vi "Reports.Results JSON V1 Data to Test Result V2 JSON.vi"(8 "File Data Objs":T7[](array[typedef]), 9 "JSON V1File":path) -> (2 "error out":errorcluster, 3 "Test Result V2":T8={"Type"="TestExec Results", "Version"="2.0.0", "TestEvent"={"ProcessStep"="", "StartTime"="", "EndTime"="", "Mode"="Production", "Operator"="", "Comment"="", "Result"={"State"="", "Code"=0, "Desc"="", "Details"=""}}, "UUTInfo"={"PN"="", "SN"="", "LotNumber"="", "DateCode"="", "AltID"="", "Properties"=[], "Revision"=""}, "Station"={"Name"="", "Location"="", "ConfigID"="", "PCName"="", "Slot"=""}, "TestSequence"={"Name"="", "Setup"=[]}, "NumericData"=[], "AttributeData"=[], "DataObjs"=[]})   [LabVIEW 2018]
uses:
  Report.Result State.ctl
  Report.Result Numeric.ctl
  Report.Result Attribute.ctl
  Report.Result DataObject.ctl
  Report.Result Data JSON V2.0.0.ctl
  Report.Result Test Event.ctl
  Report.Result Test Sequence.ctl
  Report.Result Test Station.ctl
  Results/Result XML/TestResult.Facility.ctl
  Results/Result XML/TestResult.HW Item.ctl
  Results/Result XML/TestResult.SW Item.ctl
  Results/Result XML/TestResult.Station Info.ctl
  Results/Result XML/TestResult.Test Run Info.ctl
  Results/Result XML/TestResult.Test Info.ctl
  Results/Result XML/TestResult.Symptom.State.ctl
  Results/Result XML/TestResult.Symptom.ctl
  Results/Result.Measurement and Attribute Item Status.ctl
  Results/Result XML/TestResult.UUT Result.ctl
  Results/Result XML/TestResult.FullResultData.ctl
  Report.Result UUTInfo.ctl
  Report.Result Data JSON V1_0_0.ctl
  Time/Time.Format Selector.ctl
  Results/Result.Measurement Item.ctl
  Report.Result Measurement JSON Safe.ctl
  Report.Result FileDataObject.ctl
panel:
  out "Test Result V1":T1={"Type"="Test Data", "Version"="1.0.0", "TestEvent"={"SN"="", "ProcessStep"="", "StartTime"="", "EndTime"="", "Mode"="", "Operator"="", "Comment"="", "Result"={"State"="", "Code"=0, "Desc"="", "Details"=""}}, "Station"={"Name"="", "Location"="", "ConfigID"="", "PCName"="", "Slot"=""}, "TestSequence"={"Name"="", "Setup"=[]}, "NumericData"=[], "AttributeData"=[], "DataObjs"=[]}
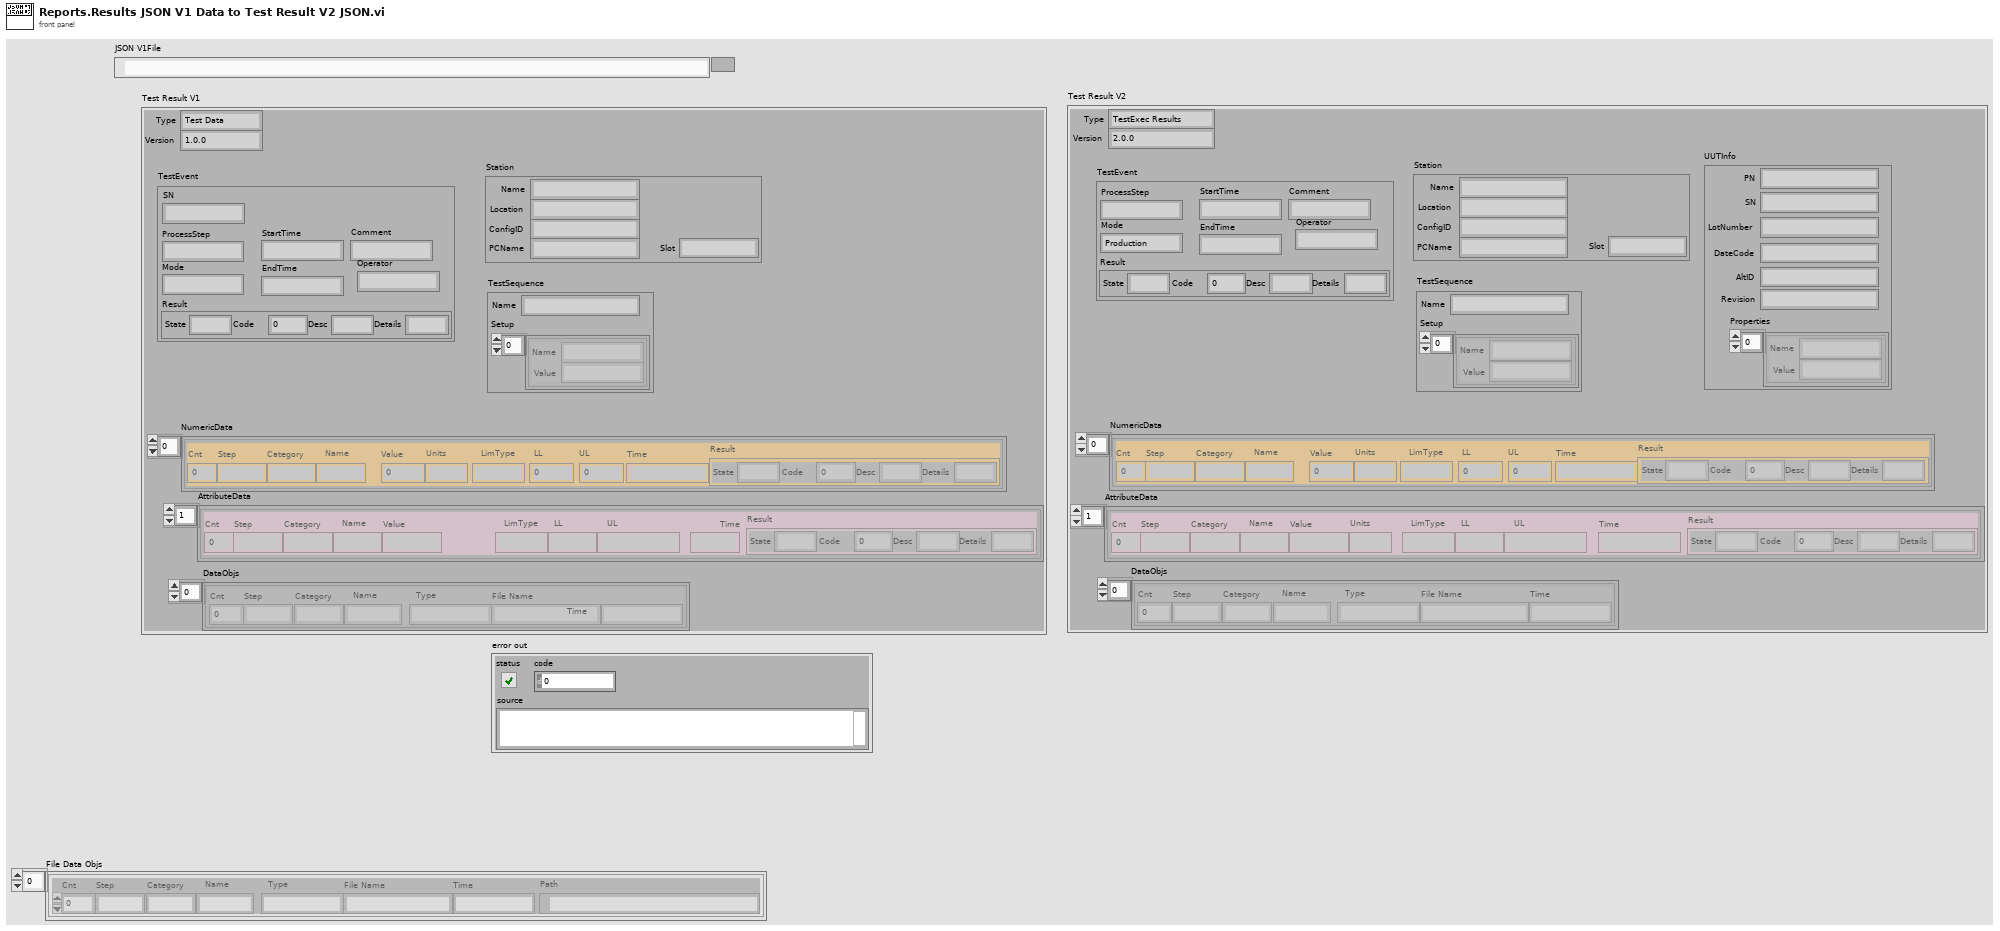
[diagram p1: front panel]
types:
  T1 = typedef "Report.Result Data JSON V1_0_0.ctl" = cluster{"Type":string, "Version":string, "TestEvent":cluster{"SN":string, "ProcessStep":string, "StartTime":string, "EndTime":string, "Mode":string, "Operator":string, "Comment":string, "Result":T2}, "Station":T3, "TestSequence":T4, "NumericData":T5[], "AttributeData":cluster{"Cnt":i32, "Step":string, "Category":string, "Name":string, "Value":string, "LimType":string, "LL":string, "UL":string, "Time":string, "Result":T2}[], "DataObjs":T6[]}
  T2 = typedef "Report.Result State.ctl" = cluster{"State":string, "Code":i32, "Desc":string, "Details":string}
  T3 = typedef "Report.Result Test Station.ctl" = cluster{"Name":string, "Location":string, "ConfigID":string, "PCName":string, "Slot":string}
  T4 = typedef "Report.Result Test Sequence.ctl" = cluster{"Name":string, "Setup":cluster{"Name":string, "Value":string}[]}
  T5 = typedef "Report.Result Numeric.ctl" = cluster{"Cnt":i32, "Step":string, "Category":string, "Name":string, "Value":dbl, "Units":string, "LimType":string, "LL":dbl, "UL":dbl, "Time":string, "Result":T2}
  T6 = typedef "Report.Result DataObject.ctl" = cluster{"Cnt":i32, "Step":string, "Category":string, "Name":string, "Type":string, "File Name":string, "Time":string}
  T7 = typedef "Report.Result FileDataObject.ctl" = cluster{"Cnt":i32, "Step":string, "Category":string, "Name":string, "Type":string, "File Name":string, "Time":string, "Path":path}
  T8 = typedef "Report.Result Data JSON V2.0.0.ctl" = cluster{"Type":string, "Version":string, "TestEvent":T9, "UUTInfo":T10, "Station":T3, "TestSequence":T4, "NumericData":T5[], "AttributeData":T11[], "DataObjs":T6[]}
  T9 = typedef "Report.Result Test Event.ctl" = cluster{"ProcessStep":string, "StartTime":string, "EndTime":string, "Mode":string, "Operator":string, "Comment":string, "Result":T2}
  T10 = typedef "Report.Result UUTInfo.ctl" = cluster{"PN":string, "SN":string, "LotNumber":string, "DateCode":string, "AltID":string, "Properties":cluster{"Name":string, "Value":string}[], "Revision":string}
  T11 = typedef "Report.Result Attribute.ctl" = cluster{"Cnt":i32, "Step":string, "Category":string, "Name":string, "Value":string, "Units":string, "LimType":string, "LL":string, "UL":string, "Time":string, "Result":T2}
  T12 = typedef "TestResult.FullResultData.ctl" = cluster{"#attributes":cluster{"Version":string}, "Facility":T13, "Station":T14, "Test Run":T17, "Test Sequence":T18, "UUTs":cluster{"UUT":T19[]}}
  T13 = typedef "TestResult.Facility.ctl" = cluster{"Name":string, "Location":string}
  T14 = typedef "TestResult.Station Info.ctl" = cluster{"Name":string, "PN":string, "SN":string, "Rev":string, "PC Name":string, "Location":string, "HW_Config":cluster{"HW_Item":T15[]}, "SW_Config":cluster{"SW_Item":T16[]}}
  T15 = typedef "TestResult.HW Item.ctl" = cluster{"Name":string, "MFG":string, "PN":string, "SN":string, "SW/FW":string, "Note":string, "Cal_ID":string, "Cal_Type":string, "Cal_Due_Date":timestamp, "Cal_Status":string}
  T16 = typedef "TestResult.SW Item.ctl" = cluster{"Name":string, "PN":string, "Version":string, "Note":string}
  T17 = typedef "TestResult.Test Run Info.ctl" = cluster{"Operator":string, "Start Time":timestamp, "Duration(s)":dbl, "Mode":string, "Comment":string, "ProcessStep":string}
  T18 = typedef "TestResult.Test Info.ctl" = cluster{"Name":string, "Config":cluster{"Config_Item":cluster{"Name":string, "Value":string}[]}}
  T19 = typedef "TestResult.UUT Info.ctl" = cluster{"Position":string, "PN":string, "SN":string, "Properties":cluster{"Property":cluster{"Name":string, "Value":string}[]}, "Result":T20, "Measurements":cluster{"Measurement":T22[]}}
  T20 = typedef "TestResult.Symptom.ctl" = cluster{"Result":T21, "Code":i32, "Description":string}
  T21 = typedef "TestResult.Symptom.State.ctl" = enum16{"Pass", "Fail", "Error", "Aborted", "Completed", "Logged"}
  T22 = typedef "Result.Measurement Item.ctl" = cluster{"Cnt":i32, "Step":string, "Category":string, "Name":string, "Value":string, "Units":string, "LimType":string, "LL":string, "UL":string, "Status":T23, "Code":i32, "Desc":string, "Time":timestamp}
  T23 = typedef "Result.Measurement and Attribute Item Status.ctl" = i32
  T24 = typedef "Time.Format Selector.ctl" = enum16{"yyyy/mm/dd HH:MM:S.sss", "yyyy-MM-ddTHH:mm:ss[.mmm]"}
  T25 = typedef "Report.Result Data JSON V2.0.0.ctl" = cluster{"Type":string, "Version":string, "TestEvent":T9, "UUTInfo":T10, "Station":T3, "TestSequence":T4, "ResultData":T26[], "DataObjs":T6[]}
  T26 = typedef "Report.Result Measurement JSON Safe.ctl" = cluster{"Cnt":i32, "Step":string, "Category":string, "Name":string, "Value":string, "Units":string, "LimType":string, "LL":string, "UL":string, "Time":string, "Result":T2}
  T27 = cluster{"SN":string, "ProcessStep":string, "StartTime":string, "EndTime":string, "Mode":string, "Operator":string, "Comment":string, "Result":T2}
  T28 = cluster{"Cnt":i32, "Step":string, "Category":string, "Name":string, "Value":string, "LimType":string, "LL":string, "UL":string, "Time":string, "Result":T2}[]
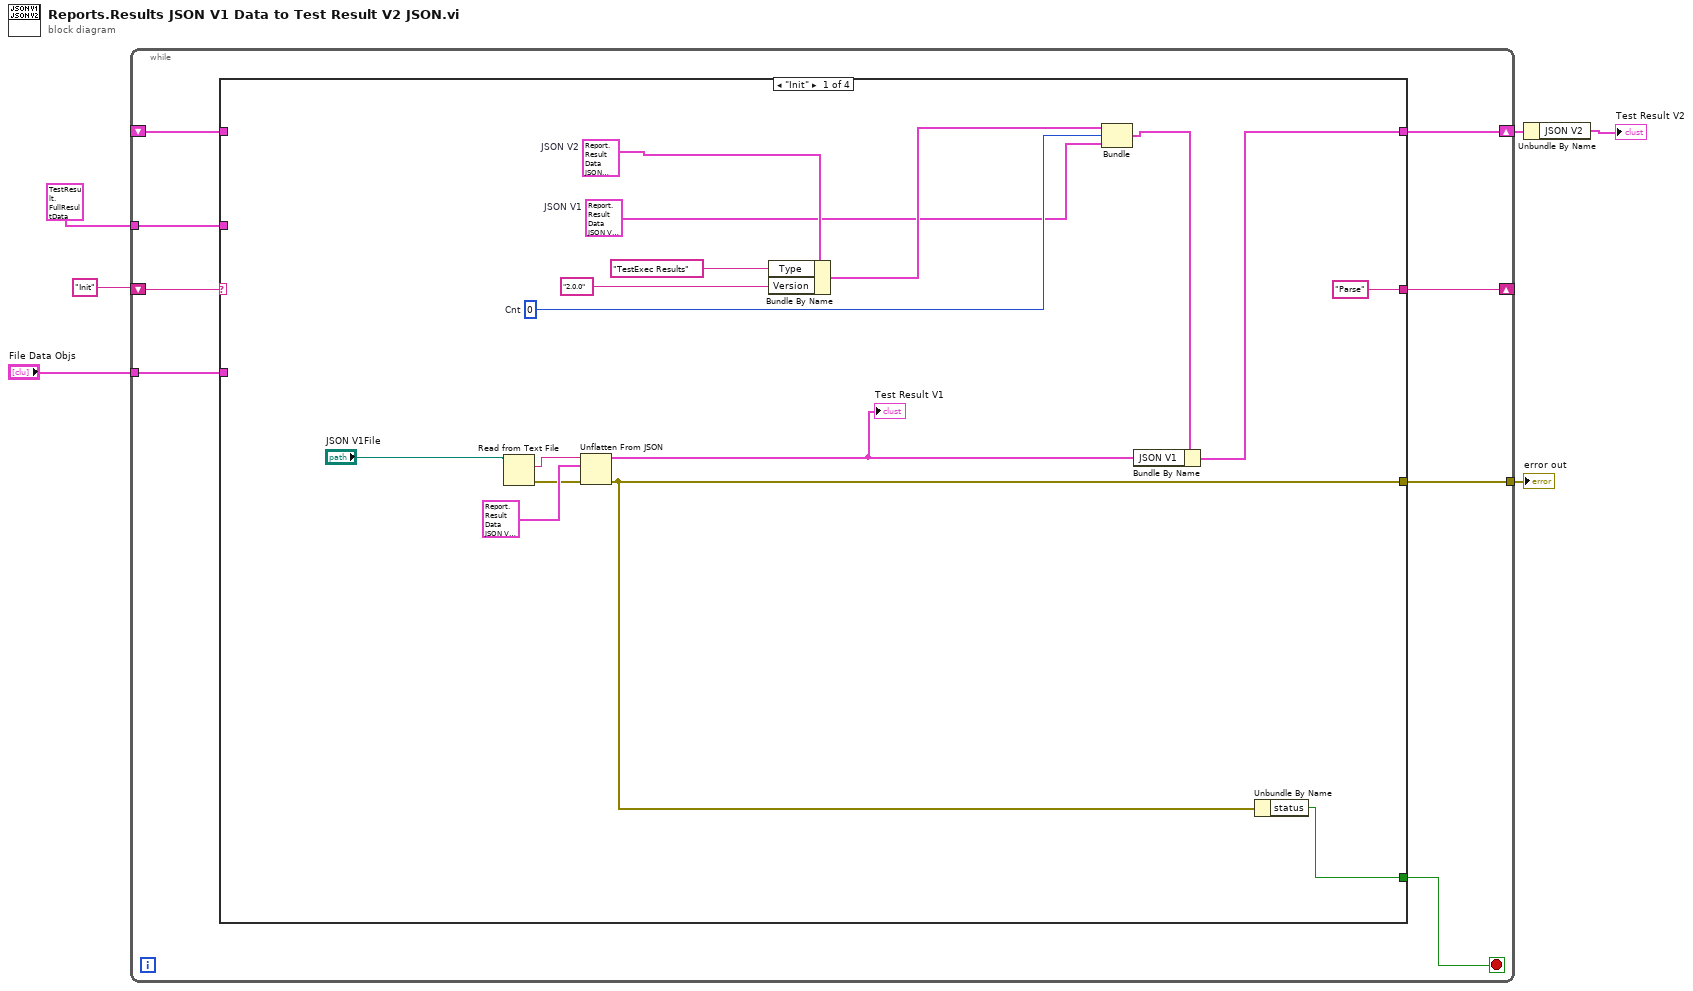
[diagram p0: block diagram]
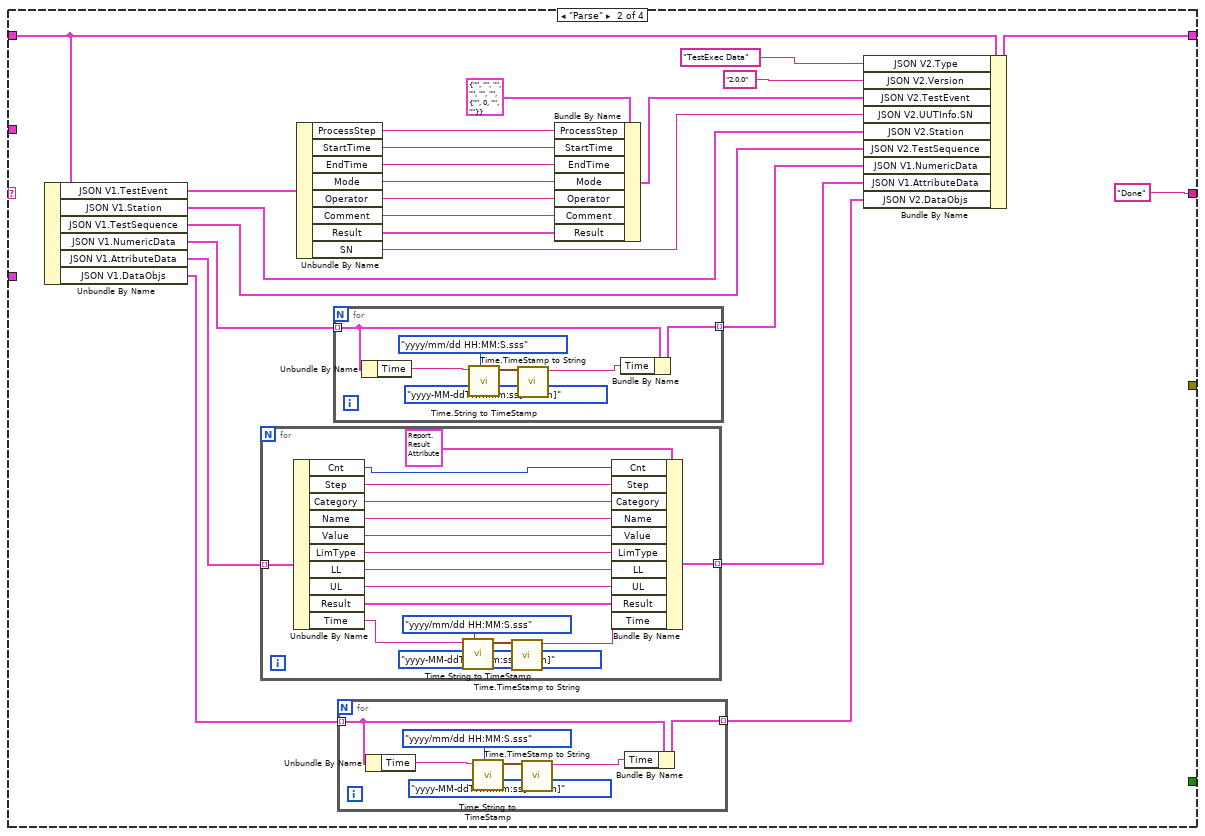
[diagram p2: hidden frame]
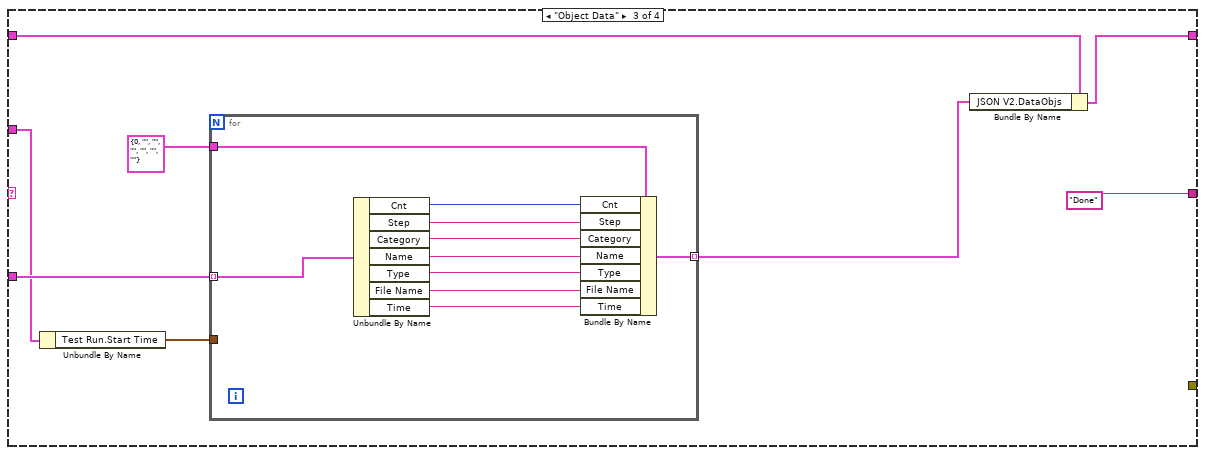
[diagram p3: hidden frame]
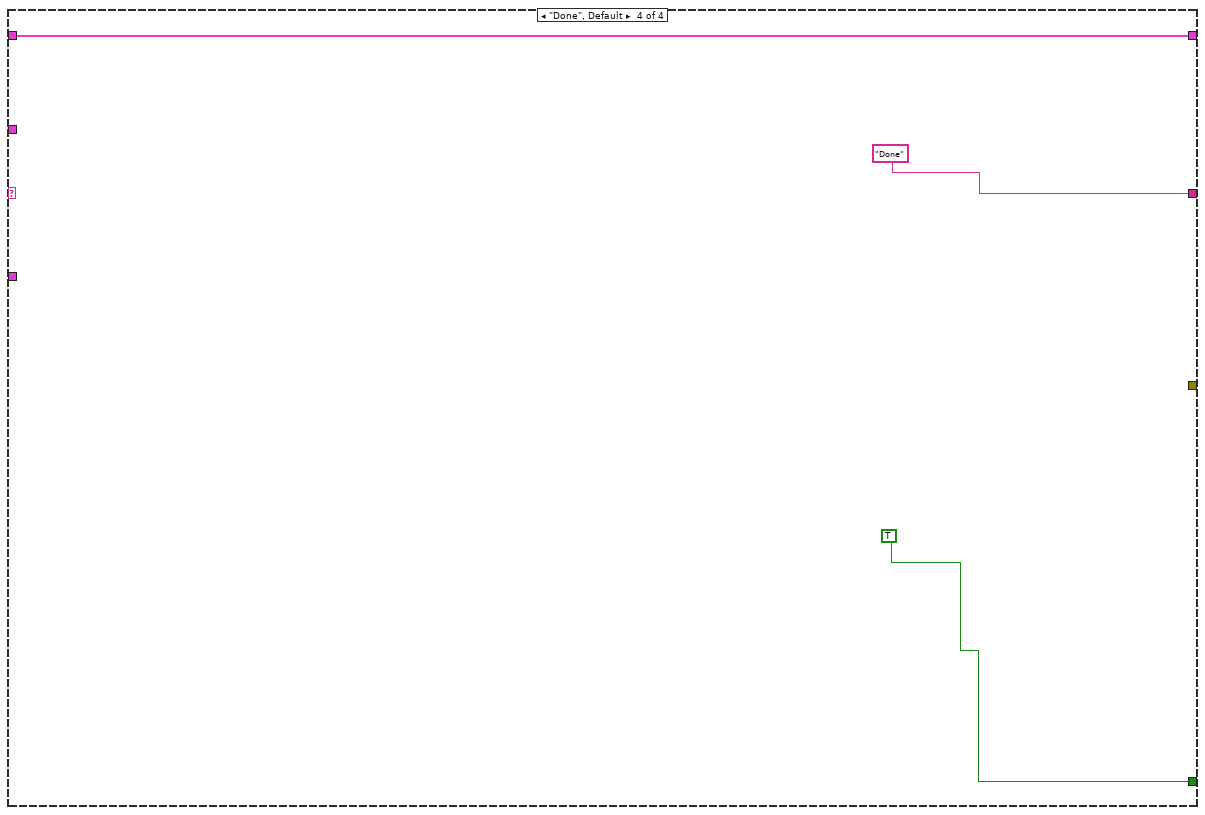
[diagram p4: hidden frame]
diagram:
  n1 = while {
    shift-right: [w8] -> w2
    shift-left: _ -> [w14]
    shift-right: [w11] -> _
    shift-left: "Init" -> [w12]
    tunnel: "File Data Objs" -> [w10]
    tunnel: T12 {"#attributes"={"Version"="MTE_1.0.0"}, "Facility"={"Name"="", "Location"=""}, "Station"={"Name"="", "PN"="", "SN"="", "Rev"="", "PC Name"="", "Location"="", "HW_Config"={"HW_Item"=[]}, "SW_Config"={"SW_Item"=[]}}, "Test Run"={"Operator"="", "Start Time"=timestamp(0 s since 1904-01-01), "Duration(s)"=0.0, "Mode"="", "Comment"="", "ProcessStep"=""}, "Test Sequence"={"Name"="", "Config"={"Config_Item"=[]}}, "UUTs"={"UUT"=[]}} ("Test Result In") -> [w9]
    tunnel: [w7] -> w1
    stop <- w13 stop-if-true
    n2 = case shown="\"Init\"" w12 {
      tunnel: w14 -> [_ w52 w87 w106]
      tunnel: [w18 w54 w93 w106] -> w8
      tunnel: [w17 _ _ TRUE] -> w13
      tunnel: ["Parse" ("Version") "Done" ("Version") "Done" ("Version") "Done"] -> w11
      tunnel: w10 -> [_ _ w89 _]
      tunnel: w9 -> [_ _ w86 _]
      tunnel: [w16 _ _ _] -> w7
      frame "Init" {
        w20 = T1 {"Type"="Test Data", "Version"="1.0.0", "TestEvent"={"SN"="", "ProcessStep"="", "StartTime"="", "EndTime"="", "Mode"="", "Operator"="", "Comment"="", "Result"={"State"="", "Code"=0, "Desc"="", "Details"=""}}, "Station"={"Name"="", "Location"="", "ConfigID"="", "PCName"="", "Slot"=""}, "TestSequence"={"Name"="", "Setup"=[]}, "NumericData"=[], "AttributeData"=[], "DataObjs"=[]}  # JSON V1
        w25 = 0  # Cnt
        w28 = T25 {"Type"="Test Data", "Version"="1.0.0", "TestEvent"={"ProcessStep"="", "StartTime"="", "EndTime"="", "Mode"="", "Operator"="", "Comment"="", "Result"={"State"="", "Code"=0, "Desc"="", "Details"=""}}, "UUTInfo"={"PN"="", "SN"="", "LotNumber"="", "DateCode"="", "AltID"="", "Properties"=[], "Revision"=""}, "Station"={"Name"="", "Location"="", "ConfigID"="", "PCName"="", "Slot"=""}, "TestSequence"={"Name"="", "Setup"=[]}, "ResultData"=[], "DataObjs"=[]}  # JSON V2
        n3 = Read from Text File(file (use dialog)="JSON V1File") -> (text=w22:string, error out=w21:errorcluster)  [unwired: 3 in, 2 out]
        n4 = Unflatten From JSON(JSON string=w22, type and defaults=T1 {"Type"="Test Data", "Version"="1.0.0", "TestEvent"={"SN"="", "ProcessStep"="", "StartTime"="", "EndTime"="", "Mode"="", "Operator"="", "Comment"="", "Result"={"State"="", "Code"=0, "Desc"="", "Details"=""}}, "Station"={"Name"="", "Location"="", "ConfigID"="", "PCName"="", "Slot"=""}, "TestSequence"={"Name"="", "Setup"=[]}, "NumericData"=[], "AttributeData"=[], "DataObjs"=[]} ("Test Result V1"), error in (no error)=w21) -> (value=w15:T1, error out=w16:errorcluster)  [unwired: 4 in]
        "Test Result V1" <- w15
        n5 = Bundle By Name(cluster=w28, "Type"="TestExec Results", "Version"="2.0.0") -> (w26:T25)
        n6 = Bundle("JSON V2"=w26, "Cnt"=w25, "JSON V1"=w20) -> (w19:cluster{"JSON V2":T25, "Cnt":i32, "JSON V1":T1})  [unwired: 1 in]
        n7 = Bundle By Name(cluster=w19, "JSON V1"=w15) -> (w18:cluster{"JSON V2":T25, "Cnt":i32, "JSON V1":T1})
        n8 = Unbundle By Name(w16) -> ("status"=w17:bool)
      }
      frame "Parse" {
        n9 = Unbundle By Name(w52) -> ("JSON V1.TestEvent"=w49:T27, "JSON V1.Station"=w38:T3, "JSON V1.TestSequence"=w37:T4, "JSON V1.NumericData"=w36:T5[], "JSON V1.AttributeData"=w34:T28, "JSON V1.DataObjs"=w33:T6[])
        n10 = for {
          tunnel: w34 -> [w78] mode=indexing
          tunnel: [w77] -> w31 mode=indexing
          n11 = Unbundle By Name(w78) -> ("Cnt"=w70:i32, "Step"=w69:string, "Category"=w68:string, "Name"=w67:string, "Value"=w66:string, "LimType"=w65:string, "LL"=w64:string, "UL"=w63:string, "Result"=w62:T2, "Time"=w72:string)
          n12 = call "Time.String to TimeStamp.vi"("TimeFormat"=Time.Format_Selector."yyyy/mm/dd HH:MM:S.sss", "Time String In"=w72) -> ("Time Stamp Out"=w76:timestamp)  [unwired: 9 in]
          n13 = call "Time.TimeStamp to String.vi"("TimeFormat"=Time.Format_Selector."yyyy-MM-ddTHH:mm:ss[.mmm]", "Time Stamp in"=w76) -> ("Time String Out"=w73:string)  [unwired: 9 in]
          n14 = Bundle By Name(cluster=T11 {"Cnt"=0, "Step"="", "Category"="", "Name"="", "Value"="", "Units"="", "LimType"="", "LL"="", "UL"="", "Time"="", "Result"={"State"="", "Code"=0, "Desc"="", "Details"=""}} ("Attribute"), "Cnt"=w70, "Step"=w69, "Category"=w68, "Name"=w67, "Value"=w66, "LimType"=w65, "LL"=w64, "UL"=w63, "Result"=w62, "Time"=w73) -> (w77:T11)
        }
        n15 = Unbundle By Name(w49) -> ("ProcessStep"=w46:string, "StartTime"=w45:string, "EndTime"=w44:string, "Mode"=w43:string, "Operator"=w42:string, "Comment"=w41:string, "Result"=w40:T2, "SN"=w39:string)
        n16 = for {
          tunnel: w36 -> [w85] mode=indexing
          tunnel: [w84] -> w35 mode=indexing
          n17 = Unbundle By Name(w85) -> ("Time"=w79:string)
          n18 = call "Time.String to TimeStamp.vi"("TimeFormat"=Time.Format_Selector."yyyy/mm/dd HH:MM:S.sss", "Time String In"=w79) -> ("Time Stamp Out"=w83:timestamp)  [unwired: 9 in]
          n19 = call "Time.TimeStamp to String.vi"("TimeFormat"=Time.Format_Selector."yyyy-MM-ddTHH:mm:ss[.mmm]", "Time Stamp in"=w83) -> ("Time String Out"=w80:string)  [unwired: 9 in]
          n20 = Bundle By Name(cluster=w85, "Time"=w80) -> (w84:T5)
        }
        n21 = for {
          tunnel: w33 -> [w61] mode=indexing
          tunnel: [w60] -> w32 mode=indexing
          n22 = Unbundle By Name(w61) -> ("Time"=w55:string)
          n23 = call "Time.String to TimeStamp.vi"("TimeFormat"=Time.Format_Selector."yyyy/mm/dd HH:MM:S.sss", "Time String In"=w55) -> ("Time Stamp Out"=w59:timestamp)  [unwired: 9 in]
          n24 = call "Time.TimeStamp to String.vi"("TimeFormat"=Time.Format_Selector."yyyy-MM-ddTHH:mm:ss[.mmm]", "Time Stamp in"=w59) -> ("Time String Out"=w56:string)  [unwired: 9 in]
          n25 = Bundle By Name(cluster=w61, "Time"=w56) -> (w60:T6)
        }
        n26 = Bundle By Name(cluster=T9 {"ProcessStep"="", "StartTime"="", "EndTime"="", "Mode"="", "Operator"="", "Comment"="", "Result"={"State"="", "Code"=0, "Desc"="", "Details"=""}} ("JSON V2.TestEvent"), "ProcessStep"=w46, "StartTime"=w45, "EndTime"=w44, "Mode"=w43, "Operator"=w42, "Comment"=w41, "Result"=w40) -> (w47:T9)
        n27 = Bundle By Name(cluster=w52, "JSON V2.Type"="TestExec Data", "JSON V2.Version"="2.0.0", "JSON V2.TestEvent"=w47, "JSON V2.UUTInfo.SN"=w39, "JSON V2.Station"=w38, "JSON V2.TestSequence"=w37, "JSON V1.NumericData"=w35, "JSON V1.AttributeData"=w31, "JSON V2.DataObjs"=w32) -> (w54:cluster{"JSON V2":T25, "Cnt":i32, "JSON V1":T1})
      }
      frame "Object Data" {
        n28 = Unbundle By Name(w86) -> ("Test Run.Start Time"=w88:timestamp)
        n29 = for {
          tunnel: w89 -> [w101] mode=indexing
          tunnel: T6 {"Cnt"=0, "Step"="", "Category"="", "Name"="", "Type"="", "File Name"="", "Time"=""} ("Data Object") -> [w103]
          tunnel: [w102] -> w91 mode=indexing
          tunnel: w88 -> [_]
          n30 = Unbundle By Name(w101) -> ("Cnt"=w100:i32, "Step"=w99:string, "Category"=w98:string, "Name"=w97:string, "Type"=w96:string, "File Name"=w95:string, "Time"=w94:string)
          n31 = Bundle By Name(cluster=w103, "Cnt"=w100, "Step"=w99, "Category"=w98, "Name"=w97, "Type"=w96, "File Name"=w95, "Time"=w94) -> (w102:T6)
        }
        n32 = Bundle By Name(cluster=w87, "JSON V2.DataObjs"=w91) -> (w93:cluster{"JSON V2":T25, "Cnt":i32, "JSON V1":T1})
      }
      frame "Done", Default {
      }
    }
  }
  "error out" <- w1
  n33 = Unbundle By Name(w2) -> ("JSON V2"=→"Test Result V2":T25)
